vi "ConvertDMS2DD.vi"(8 "error in":errorcluster, 9 "Seconds":dbl, 10 "Minutes":dbl, 11 "Degrees":dbl) -> (0 "error out":errorcluster, 3 "Degree Decimal":dbl format="%.6f")   [LabVIEW 2010]
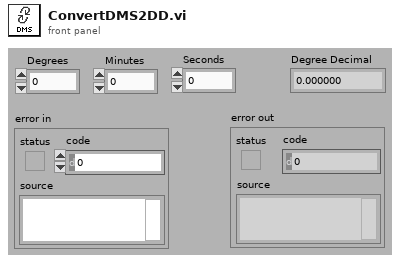
[diagram p1: front panel]
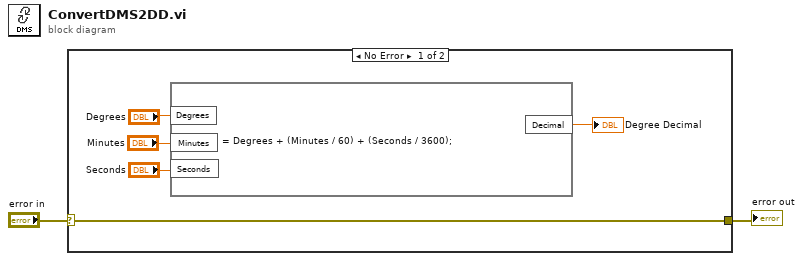
[diagram p0: block diagram]
diagram:
  n1 = case shown="No Error" "error in" {
    selector: "error in" -> [w3 w8]
    tunnel: [w3 w8] -> w1
    frame No Error {
      n2 = formula code="Decimal = Degrees + (Minutes / 60) + (Seconds / 3600);"("Degrees"="Degrees", "Minutes"="Minutes", "Seconds"="Seconds") -> ("Decimal"=→"Degree Decimal":dbl)
    }
    frame Error {
    }
  }
  "error out" <- w1
